vi "Get Total Column Number.vi"(8 "error in (no error)":errorcluster, 11 "Scan Driver.lvclass":refnum<class "Scan Driver.lvclass">) -> (0 "error out":errorcluster, 2 "# of Columns":i32, 3 "Scan Driver.lvclass":refnum<class "Scan Driver.lvclass">)   [LabVIEW 2023, in "Scan Driver.lvclass"]
uses:
  Scan Driver.lvclass
  Scan Driver.lvclass/Scan Driver.ctl
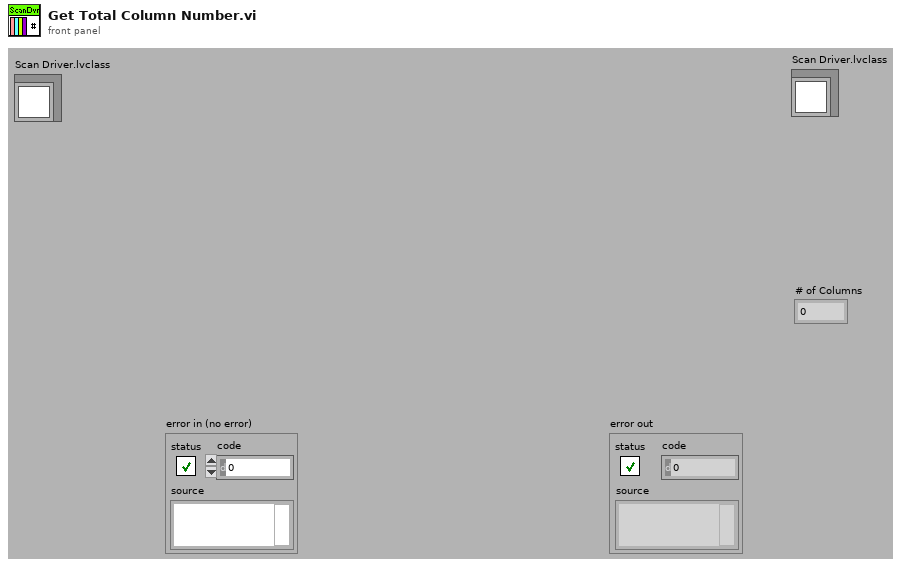
[diagram p1: front panel]
types:
  T1 = typedef "Readable.lvclass/Data Store.ctl" = T2[][]
  T2 = typedef "Readable.lvclass/Data Point.ctl" = cluster{"t":T3, "x":T4}
  T3 = typedef "Readable.lvclass/Time.ctl" = timestamp
  T4 = typedef "Readable.lvclass/X.ctl" = dbl
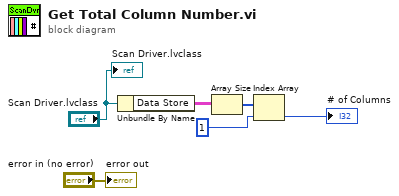
[diagram p0: block diagram]
diagram:
  n1 = Unbundle By Name("Scan Driver.lvclass") -> ("Data Store"=w4:T1)
  n2 = Array Size(array=w4) -> (size(s)=w3:i32[])
  n3 = Index Array(array=w3, index=1) -> (element=→"# of Columns":i32)
  "Scan Driver.lvclass" <- "Scan Driver.lvclass"
  "error out" <- "error in (no error)"
